vi "Append eol.vi"(1 "INPUT STRING":string) -> (0 "OUTPUT STRING (PLUS End of Line)":string)   [LabVIEW 2018]
doc: "Concatenates a Carriage Return [CR ] at the end of the input string. Copyright Laouris & Reinking, May 89"
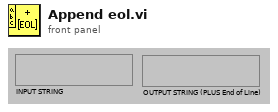
[diagram p1: front panel]
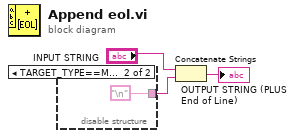
[diagram p0: block diagram]
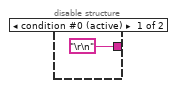
[diagram p2: hidden frame]
diagram:
  n1 = disable-structure shown="TARGET_TYPE==Mac" {
    disable-tunnel: ["\r\n" "\n"] -> w1
    frame condition #0 (active) {
    }
    frame condition #1 {
    }
  }
  n2 = Concatenate Strings("INPUT STRING", w1) -> (→"OUTPUT STRING (PLUS End of Line)":string)
